vi "cRIO All Modules Main.vi"() -> ()   [LabVIEW 2014]
doc: "This application launches and executes the Tag Bus Data framework configuration for the specified target alias. This is a simple example of the framework API functions, but may also be a suitable starting point for a Host UI or Thick Client that is running a local version of the framework."
uses:
  <vilib>/NI/Module Execution Interface/Engine Runtime/Execution States.ctl
  <vilib>/NI/Module Execution Interface/Engine Runtime/Fault.ctl
  <vilib>/NI/Tag Bus Module Framework/runtime/error classification.ctl
  <vilib>/userdefined/High Color/nirio_resource_hc.ctl
  <vilib>/NI/Module Execution Interface/Engine Runtime/Engine Runtime Interface.lvclass
  <vilib>/NI/DCAF/Tag Editor Core/Framework Configuration Classes/target runtime/PL_Target Runtime.lvclass
  <vilib>/NI/Tag Bus Module Framework/FPGA manager/FPGA manager.lvlib
  <vilib>/rvi/interface/nirviOpenFPGA/nirviOpenFPGA.xnode
  <vilib>/NI/Tag Bus Module Framework/FPGA manager/methods.ctl
  <vilib>/NI/Tag Bus Module Framework/runtime/TBM module execution interface.lvclass
panel:
  in  "configuration file path":path=path "C:/Users/bsnover/Desktop/DCAF Integration Testing/Testing Project/Integration Testing Configuration.pcfg"
  in  "target alias":string="cRIO Integration"
  out "engine status":T4(array[cluster])
  in  "stop":bool
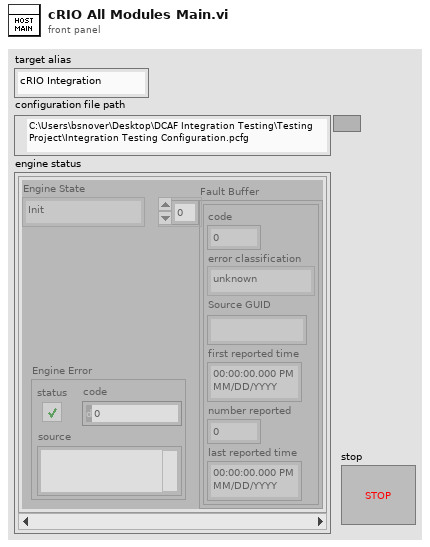
[diagram p1: front panel]
types:
  T1 = typedef "Engine Runtime Interface.lvclass/Execution States.ctl" = enum16{"Init", "Pre-Operational", "Safe-Operational", "Operational", "Stopped"}
  T2 = typedef "Engine Runtime Interface.lvclass/Fault.ctl" = cluster{"code":i32, "error classification":T3, "Source GUID":string, "first reported time":timestamp, "number reported":u32, "last reported time":timestamp}
  T3 = typedef "TBM module execution interface.lvclass/error classification.ctl" = enum16{"unknown", "none", "trivial", "recoverable", "critical"}
  T4 = cluster{"Engine State":T1, "Fault Buffer":T2[], "Engine Error":errorcluster}[]
  T5 = typedef "FPGA manager.lvlib/methods.ctl" = enum16{"initialize bitfile", "cache bitfile", "locate bitfile", "close bitfile", "clear manager"}
  T6 = typedef "nirio_resource_hc.ctl" = tag
  T7 = cluster{"Engine State":T1, "faults":T2[], "Engine Error":errorcluster}
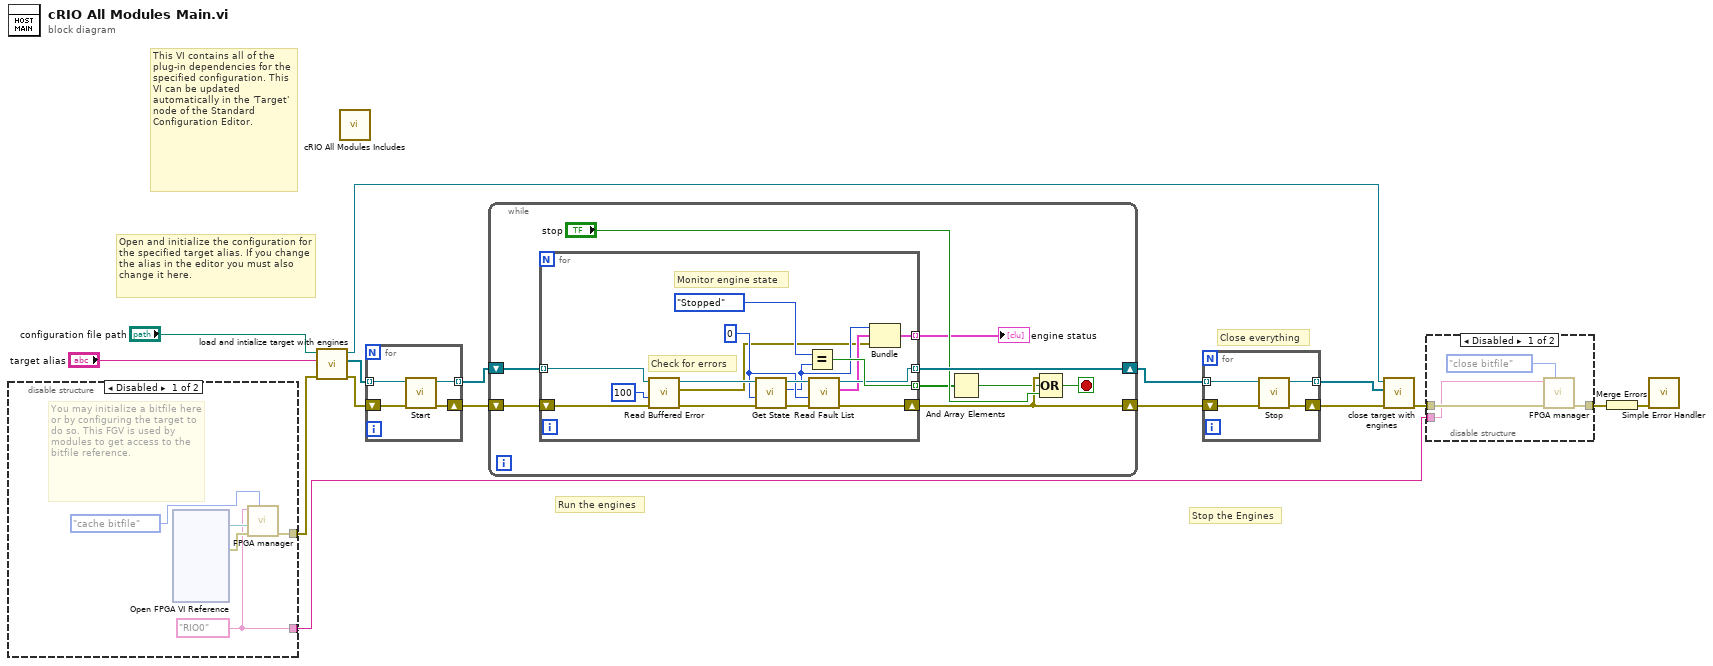
[diagram p0: block diagram]
diagram:
  # "Open and initialize the configuration for the specified target alias. If you change the alias in the editor you must also change it here."
  # "Close everything"
  # "Stop the Engines"
  # "This VI contains all of the plug-in dependencies for the specified configuration. This VI can be updated automatically in the 'Target' node of the Standard Configuration Editor."
  # "Run the engines"
  n1 = disable-structure shown="Disabled" {
    disable-tunnel: [w21 _] -> w6
    disable-tunnel: [w17 _] -> w5
    frame Disabled {
      w17 = T6 "RIO0" ("RIO resource")
      # "You may initialize a bitfile here or by configuring the target to do so. This FGV is used by modules to get access to the bitfile reference."
      n2 = xnode "Open FPGA VI Reference"() -> ("FPGA VI Reference Out"=w19:refnum<k20>, "error out"=w20:errorcluster)  [unwired: 2 in]
      n3 = call <vilib>:"FPGA manager.vi"("action"=methods."cache bitfile", "error in"=w20, "bitfile to cache"=w19, "RIO resource"=w17) -> ("error out"=w21:errorcluster)  [unwired: 5 in, 2 out]
    }
    frame Enabled {
    }
  }
  n4 = call <vilib>:"load and intialize target with engines.vi"("error in"=w6, "target alias"="target alias", "file path"="configuration file path") -> ("error out"=w13:errorcluster, "engine runtime interfaces"=w12:refnum<class "Engine Runtime Interface.lvclass">[], "target runtime"=w9:refnum<class "PL_Target Runtime.lvclass">)  [unwired: 6 in]
  n5 = call "cRIO All Modules Includes.vi"() -> ()  [unwired: 12 in]
  n6 = for {
    tunnel: [w25] -> w16 mode=indexing
    tunnel: w12 -> [w22] mode=indexing
    shift-right: [w24] -> w1
    shift-left: w13 -> [w23]
    n7 = call-dynamic "Start.vi"("error in"=w23, "Engine Runtime Interface in"=w22) -> ("error out"=w24:errorcluster, "Engine Runtime Interface out"=w25:refnum<class "Engine Runtime Interface.lvclass">)  [unwired: 8 in]
  }
  n8 = while {
    shift-right: [w32] -> w15
    shift-left: w16 -> [w34]
    shift-right: [w29] -> w14
    shift-left: w1 -> [w33]
    stop <- w30 stop-if-true
    n9 = for {
      tunnel: w34 -> [w50] mode=indexing
      tunnel: [w41] -> w32 mode=indexing
      tunnel: [w45] -> w27 mode=indexing
      shift-right: [w40] -> w29
      shift-left: w33 -> [w49]
      tunnel: [w35] -> w28 mode=indexing
      w39 = 0 ("timeout (-1)")
      # "Monitor engine state"
      # "Check for errors"
      n10 = call-dynamic "Read Buffered Error.vi"("error in"=w49, "timeout in ms (0)"=100, "Engine Runtime Interface in"=w50) -> ("error out"=w47:errorcluster, "Engine Error"=w36:errorcluster, "Engine Runtime Interface out"=w48:refnum<class "Engine Runtime Interface.lvclass">)  [unwired: 6 in]
      n11 = call-dynamic "Get State.vi"("error in"=w47, "timeout (-1)"=w39, "Engine Runtime Interface in"=w48) -> ("error out"=w43:errorcluster, "Engine State"=w38:T1, "Engine Runtime Interface out"=w42:refnum<class "Engine Runtime Interface.lvclass">)  [unwired: 6 in]
      n12 = Equal?(x=Execution_States."Stopped" ("Engine State"), y=w38) -> (x = y?=w45:bool)
      n13 = call-dynamic "Read Fault List.vi"("error in"=w43, "timeout (-1)"=w39, "Engine Runtime Interface in"=w42) -> ("error out"=w40:errorcluster, "faults"=w37:T2[], "Engine Runtime Interface out"=w41:refnum<class "Engine Runtime Interface.lvclass">)  [unwired: 6 in]
      n14 = Bundle("Engine State"=w38, "faults"=w37, "Engine Error"=w36) -> (w35:T7)  [unwired: 1 in]
    }
    "engine status" <- w28
    n15 = And Array Elements(Boolean array=w27) -> (logical AND=w26:bool)
    n16 = Compound Arithmetic op=OR(w29, w26, "stop") -> (w30:bool)
  }
  n17 = for {
    tunnel: w15 -> [w54] mode=indexing
    shift-right: [w51] -> w8
    shift-left: w14 -> [w53]
    tunnel: [w52] -> w10 mode=indexing
    n18 = call-dynamic "Stop.vi"("error in"=w53, "Engine Runtime Interface in"=w54) -> ("error out"=w51:errorcluster, "Engine Runtime Interface out"=w52:refnum<class "Engine Runtime Interface.lvclass">)  [unwired: 8 in]
  }
  n19 = call <vilib>:"close target with engines.vi"("error in"=w8, "Engine Runtime Interfaces"=w10, "Target Runtime"=w9) -> ("error out"=w4:errorcluster)  [unwired: 8 in]
  n20 = disable-structure shown="Disabled" {
    disable-tunnel: [w57 w59] -> w3
    disable-tunnel: w4 -> [w58 w59]
    disable-tunnel: w5 -> [w55 _]
    frame Disabled {
      n21 = call <vilib>:"FPGA manager.vi"("action"=methods."close bitfile", "error in"=w58, "RIO resource"=w55) -> ("error out"=w57:errorcluster)  [unwired: 6 in, 2 out]
    }
    frame Enabled {
    }
  }
  n22 = Merge Errors(w3) -> (w2:errorcluster)
  n23 = call <vilib>:"Simple Error Handler.vi"("error in (no error)"=w2) -> ()  [unwired: 4 in, 5 out]
